vi "Populate Response Variable - Advance.vi"(5 "Variant":variant, 6 "Error in":errorcluster caption="Error in (no error)", 7 "depth":i32, 8 "variable History":string[](array[string]), 9 "String might with variables":string) -> (0 "Error out":errorcluster, 3 "String out":string, 4 "Variant Out":variant)   [LabVIEW 2020]
uses:
  <userlib>/_NEVSTOP/Communicable State Machine(CSM)/addons/INI-Static-Variable-Support/INI-Static-Variable-Support.lvlib
  <userlib>/_NEVSTOP/Communicable State Machine(CSM)/_Shared/CSM Shared.lvlib
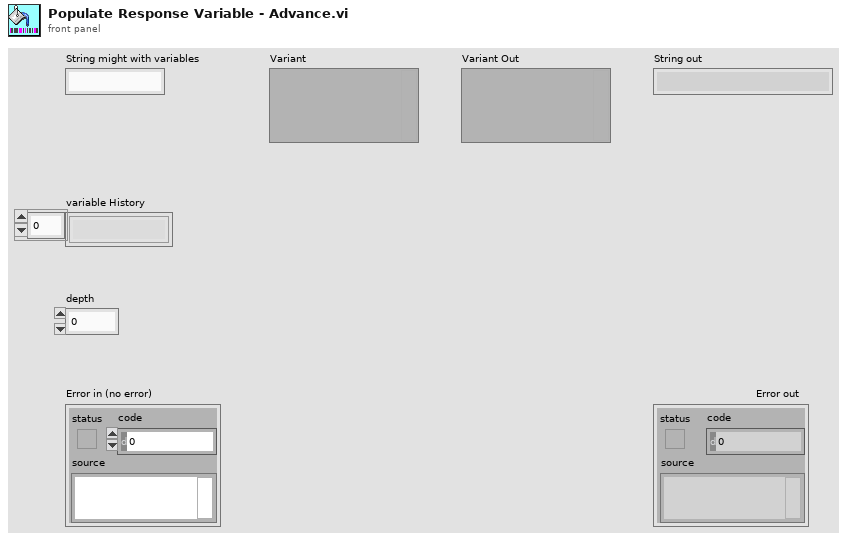
[diagram p1: front panel]
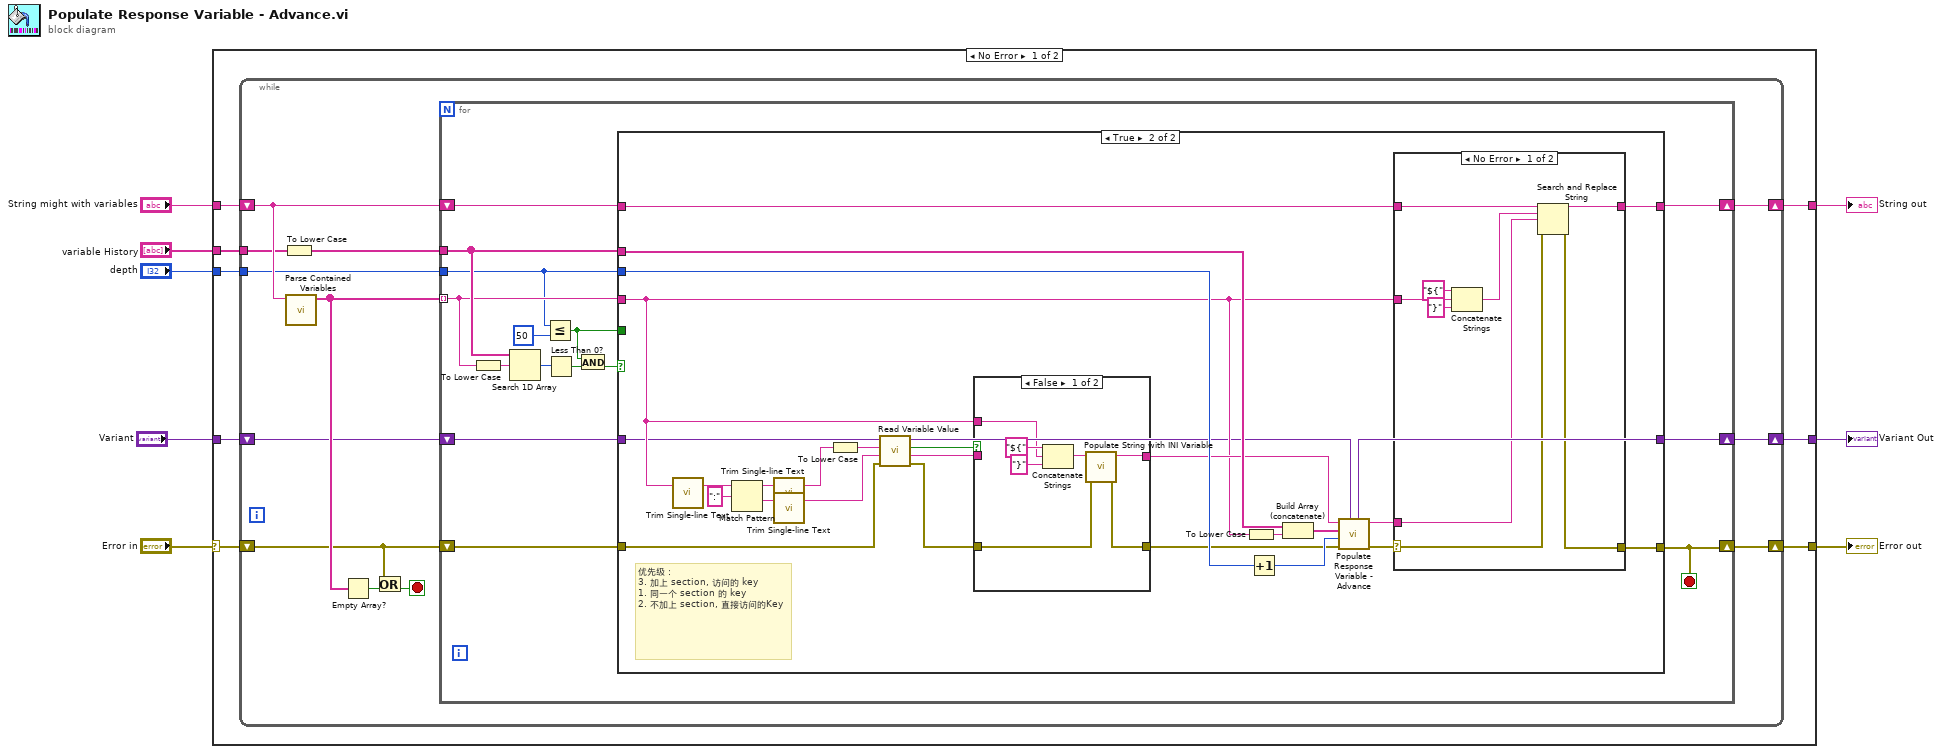
[diagram p0: block diagram]
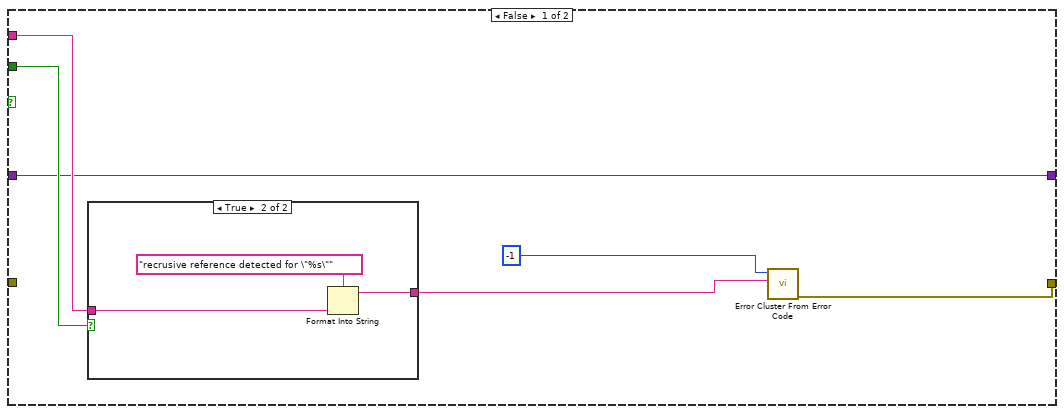
[diagram p2: hidden frame]
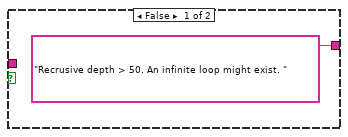
[diagram p3: hidden frame]
diagram:
  n1 = case shown="No Error" "Error in" {
    selector: "Error in" -> [w13 w102]
    tunnel: [w16 w101] -> w8
    tunnel: "String might with variables" -> [w15 w101]
    tunnel: [w12 w102] -> w5
    tunnel: "variable History" -> [w14 _]
    tunnel: "depth" -> [w11 _]
    tunnel: "Variant" -> [w10 w100]
    tunnel: [w9 w100] -> w1
    frame No Error {
      n2 = while {
        shift-right: [w28] -> w16
        shift-left: w15 -> [w26]
        tunnel: w14 -> [w23]
        shift-right: [w24] -> w12
        shift-left: w13 -> [w20]
        tunnel: w11 -> [w19]
        shift-right: [w17] -> w9
        shift-left: w10 -> [w18]
        stop <- w21 stop-if-true
        n3 = To Lower Case(string=w23) -> (all lower case string=w22:string[])
        n4 = call <userlib>:"Parse Contained Variables.vi"("String"=w26) -> ("Contained Variables"=w25:string[])  [unwired: 10 in]
        n5 = Empty Array?(array=w25) -> (empty?=w27:bool)
        n6 = Or(x=w20, y=w27) -> (x .or. y?=w21:bool)
        n7 = for {
          tunnel: w25 -> [w40] mode=indexing
          shift-right: [w42] -> w28
          shift-left: w26 -> [w43]
          tunnel: w22 -> [w41]
          shift-right: [w37] -> w24
          shift-left: w20 -> [w36]
          tunnel: w19 -> [w34]
          shift-right: [w29] -> w17
          shift-left: w18 -> [w30]
          stop <- w37 stop-if-true
          n8 = To Lower Case(string=w40) -> (all lower case string=w39:string)
          n9 = Search 1D Array(1D array=w41, element=w39) -> (index of element=w38:i32)  [unwired: 1 in]
          n10 = Less Or Equal?(x=w34, y=50) -> (x <= y?=w32:bool)
          n11 = Less Than 0?(x=w38) -> (x < 0?=w31:bool)
          n12 = And(x=w32, y=w31) -> (x .and. y?=w35:bool)
          n13 = case shown="True" w35 {
            tunnel: w43 -> [_ w80]
            tunnel: [_ w79] -> w42
            tunnel: [w49 w78] -> w37
            tunnel: w41 -> [_ w68]
            tunnel: w40 -> [w47 w59]
            tunnel: w36 -> [_ w64]
            tunnel: w34 -> [_ w66]
            tunnel: w32 -> [w45 _]
            tunnel: w30 -> [w44 w58]
            tunnel: [w44 w63] -> w29
            frame False {
              n14 = case shown="True" w45 {
                tunnel: w47 -> [_ w52]
                tunnel: ["Recrusive depth > 50. An infinite loop might exist. " w51] -> w46
                frame False {
                }
                frame True {
                  n15 = Format Into String(format string="recrusive reference detected for \"%s\"", w52) -> (resulting string=w51:string)  [unwired: 2 in, 1 out]
                }
              }
              n16 = call <vilib>:"Error Cluster From Error Code.vi"("error message (\"\")"=w46, "error code (0)"=-1 ("code")) -> ("error out"=w49:errorcluster)  [unwired: 7 in]
            }
            frame True {
              # "优先级：\n3. 加上 section, 访问的 key \n1. 同一个 section 的 key\n2. 不加上 section, 直接访问的Key"
              n17 = call <userlib>:"Trim Single-line Text.vi"("single-line text"=w59) -> ("trimed text"=w73:string)  [unwired: 2 in]
              n18 = Match Pattern(string=w73, regular expression=":") -> (before substring=w76:string, after substring=w75:string)  [unwired: 1 in, 2 out]
              n19 = call <userlib>:"Trim Single-line Text.vi"("single-line text"=w76) -> ("trimed text"=w70:string)  [unwired: 2 in]
              n20 = call <userlib>:"Trim Single-line Text.vi"("single-line text"=w75) -> ("trimed text"=w74:string)  [unwired: 2 in]
              n21 = To Lower Case(string=w70) -> (all lower case string=w57:string)
              n22 = call "Read Variable Value.vi"("error in (no error)"=w64, "Default Value"=w74, "String"=w57, "Variant in"=w58) -> ("error out"=w61:errorcluster, "Value"=w55:string, "Found"=w56:bool, "Variant out"=w54:variant)  [unwired: 4 in]
              n23 = case shown="False" w56 {
                tunnel: w55 -> [_ w89]
                tunnel: [w85 w89] -> w62
                tunnel: w61 -> [w87 w88]
                tunnel: [w86 w88] -> w60
                tunnel: w59 -> [w81 _]
                frame False {
                  n24 = Concatenate Strings("${" ("regular expression"), w81, "}" ("regular expression")) -> (w82:string)
                  n25 = call <userlib>:"Populate String with INI Variable.vi"("Error in"=w87, "String might with variables"=w82) -> ("Error out"=w86:errorcluster, "String out"=w85:string)  [unwired: 6 in]
                }
                frame True {
                }
              }
              n26 = To Lower Case(string=w59) -> (all lower case string=w67:string)
              n27 = Increment(x=w66) -> (x+1=w65:i32)
              n28 = Build Array (concatenate)(w68, w67) -> (w69:string[])
              n29 = call "Populate Response Variable - Advance.vi"("Variant"=w54, "Error in"=w60, "depth"=w65, "variable History"=w69, "String might with variables"=w62) -> ("Error out"=w71:errorcluster, "String out"=w72:string, "Variant Out"=w63:variant)  [unwired: 2 in]
              n30 = case shown="No Error" w71 {
                selector: w71 -> [w92 w99]
                tunnel: w80 -> [w96 _]
                tunnel: [w95 _] -> w79
                tunnel: [w94 w99] -> w78
                tunnel: w72 -> [w93 _]
                tunnel: w59 -> [w90 _]
                frame No Error {
                  n31 = Concatenate Strings("${" ("regular expression"), w90, "}" ("regular expression")) -> (w91:string)
                  n32 = Search and Replace String(input string=w96, search string=w91, replace string=w93, error in=w92) -> (result string=w95:string, error out=w94:errorcluster)  [unwired: 4 in, 2 out]
                }
                frame Error {
                }
              }
            }
          }
        }
      }
    }
    frame Error {
    }
  }
  "String out" <- w8
  "Error out" <- w5
  "Variant Out" <- w1
